vi "event_disconnected.vi"(11 "message":string) -> ()   [LabVIEW 2014]
uses:
  QwaveSys_ESP8266/QwaveSys_ESP8266.lvlib
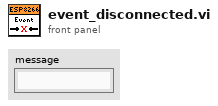
[diagram p1: front panel]
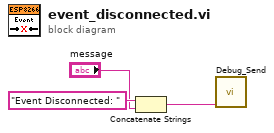
[diagram p0: block diagram]
diagram:
  n1 = Concatenate Strings("Event Disconnected: " ("string"), "message") -> (w1:string)
  n2 = call "Debug_Send.vi"("DATA"=w1) -> ()  [unwired: 11 in]
